vi "TIO RPC Verify.vi"(8 "error in (no error)":errorcluster, 9 "Starts With":string="Twinleaf VM", 10 "Topic":string="mcu.desc", 11 "TS Connection":T1={"Type"=enum."TCP", "Serial"="serial:///dev/cu.usbserial-00000", "TCP"=refnum, "Timeout"=500}) -> (0 "error out":errorcluster={"status"=TRUE, "code"=-1073807252, "source"="VISA Read in SLIP Decode Serial Read.vi->NN VISA Read.vi->NN RPC.vi"}, 1 "Respose":string, 2 "Verify":bool, 3 "TS Connection":T1={"Type"=enum."TCP", "Serial"="serial:///dev/cu.usbserial-00000", "TCP"=refnum, "Timeout"=500})   [LabVIEW 2016]
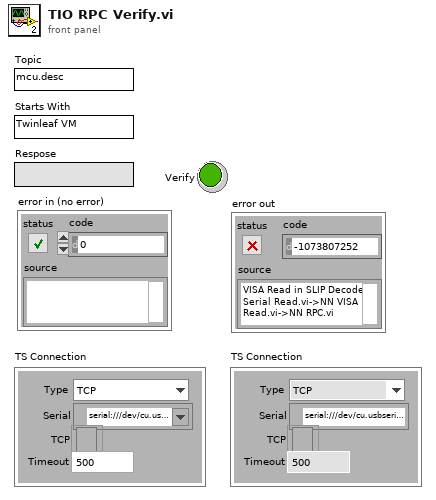
[diagram p1: front panel]
types:
  T1 = cluster{"Type":enum16{"TCP", "Serial"}, "Serial":refnum<visa-resource-name>, "TCP":refnum<k5>, "Timeout":u32}
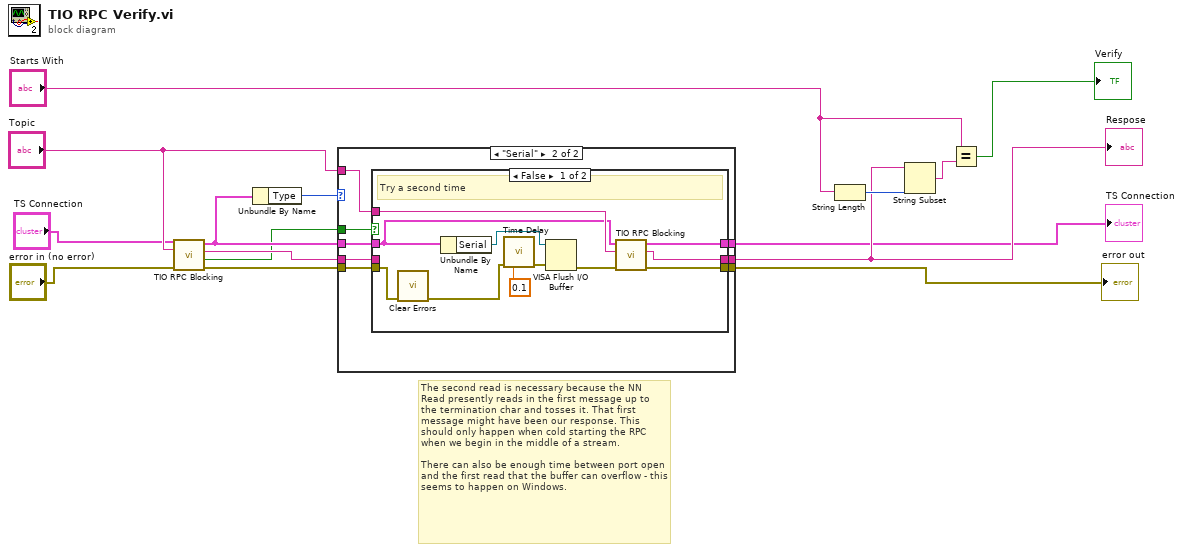
[diagram p0: block diagram]
diagram:
  # "The second read is necessary because the NN Read presently reads in the first message up to the termination char and tosses it. That first message might have been our response. This should only happen when cold starting the RPC when we begin in the middle of a stream.\n\nThere can also be enough time between port open and the first read that the buffer can overflow - this seems to happen on Windows."
  n1 = call "TIO RPC Blocking.vi"("error in (no error)"="error in (no error)", "Named Method"="Topic", "TS Connection"="TS Connection") -> ("error out"=w8:errorcluster, "Response"=w1:bool, "Respose"=w2:string, "TS Connection"=w3:T1)  [unwired: 5 in]
  n2 = Unbundle By Name(w3) -> ("Type"=w4:enum16{"TCP", "Serial"})
  n3 = case shown="\"Serial\"" w4 {
    tunnel: w1 -> [_ w26]
    tunnel: w3 -> [w18 w25]
    tunnel: w2 -> [w17 w24]
    tunnel: [w16 w23] -> w10
    tunnel: [w18 w22] -> w5
    tunnel: [w17 w21] -> w9
    tunnel: w8 -> [w16 w20]
    tunnel: "Topic" -> [_ w19]
    frame "TCP" {
    }
    frame "Serial" {
      n4 = case shown="False" w26 {
        tunnel: w25 -> [w28 w40]
        tunnel: w24 -> [_ w38]
        tunnel: w20 -> [w32 w39]
        tunnel: [w37 w39] -> w23
        tunnel: [w36 w40] -> w22
        tunnel: [w27 w38] -> w21
        tunnel: w19 -> [w30 _]
        frame False {
          # "Try a second time"
          n5 = call <vilib>:"Clear Errors.vi"("error in (no error)"=w32) -> ("error out"=w31:errorcluster)  [unwired: 5 in, 1 out]
          n6 = Unbundle By Name(w28) -> ("Serial"=w29:refnum<visa-resource-name>)
          n7 = call "Time Delay"("error in (no error)"=w31, "Delay Time (s)"=0.1) -> ("error out"=w35:errorcluster)  [unwired: 9 in]
          n8 = VISA Flush I/O Buffer(VISA resource name=w29, error in (no error)=w35) -> (error out=w34:errorcluster)  [unwired: 1 in, 1 out]
          n9 = call "TIO RPC Blocking.vi"("error in (no error)"=w34, "Named Method"=w30, "TS Connection"=w28) -> ("error out"=w37:errorcluster, "Respose"=w27:string, "TS Connection"=w36:T1)  [unwired: 5 in, 1 out]
        }
        frame True {
        }
      }
    }
  }
  "error out" <- w10
  "Respose" <- w9
  "TS Connection" <- w5
  n10 = String Length(string="Starts With") -> (length=w14:i32)
  n11 = String Subset(string=w9, length (rest)=w14) -> (substring=w12:string)  [unwired: 1 in]
  n12 = Equal?(x="Starts With", y=w12) -> (x = y?=→"Verify":bool)
